vi "ProcessCANWrite.vi"(6 "Write Values":sgl[](array[numeric]), 8 "error in (no error)":errorcluster, 10 "Queue in":refnum<queue>, 11 "WriteFramesInfo":T1(array[cluster])) -> (0 "error out":errorcluster, 2 "WriteFramesSize":i32, 4 "Write Values":sgl[](array[numeric]))   [LabVIEW 2016, in "DSI-RT.lvlib"]
uses:
  DSI-RT.lvlib
  <vilib>/RioEmbeddedCAN/RioEmbeddedCAN.llb/CANFrameControl.ctl
  <vilib>/addons/Software Calibration Management/xSCM/Get/Get Variant.vi
  <vilib>/addons/Software Calibration Management/xSCM/SCM-API.lvlib
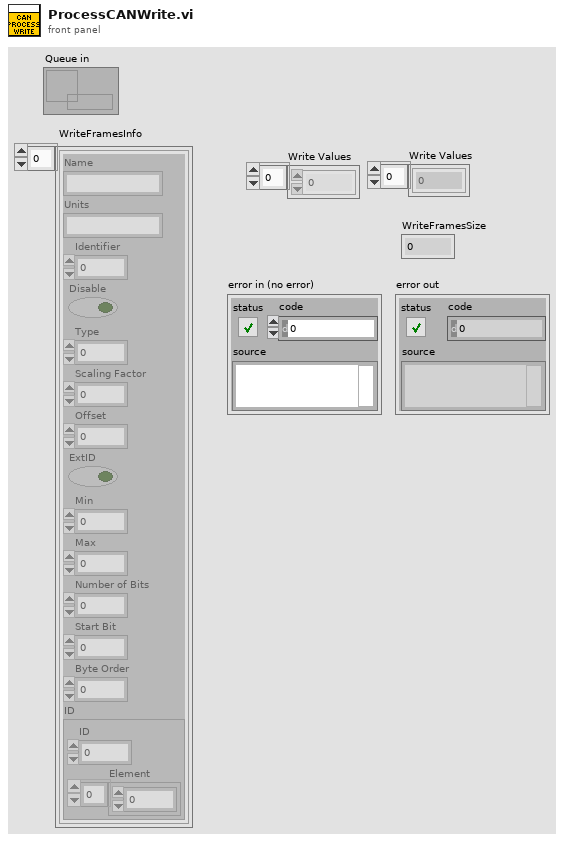
[diagram p1: front panel]
types:
  T1 = cluster{"Name":string, "Units":string, "Identifier":u32, "Disable":bool, "Type":u16, "Scaling Factor":sgl, "Offset":sgl, "ExtID":bool, "Min":sgl, "Max":sgl, "Number of Bits":u8, "Start Bit":u8, "Byte Order":u8, "ID":cluster{"ID":u32, "Element":i32[]}}[]
  T2 = cluster{"StartBit":u8, "Num Bits":u8, "Byte Order":u8, "Data Type":u8}
  T3 = cluster{"ScalingFactor":sgl, "Offset":sgl, "Maximum":sgl, "Minimum":sgl}
  T4 = typedef "CANFrameControl.ctl" = cluster{"identifier":u32, "extended?":bool, "type":u8, "payload":u8[]}
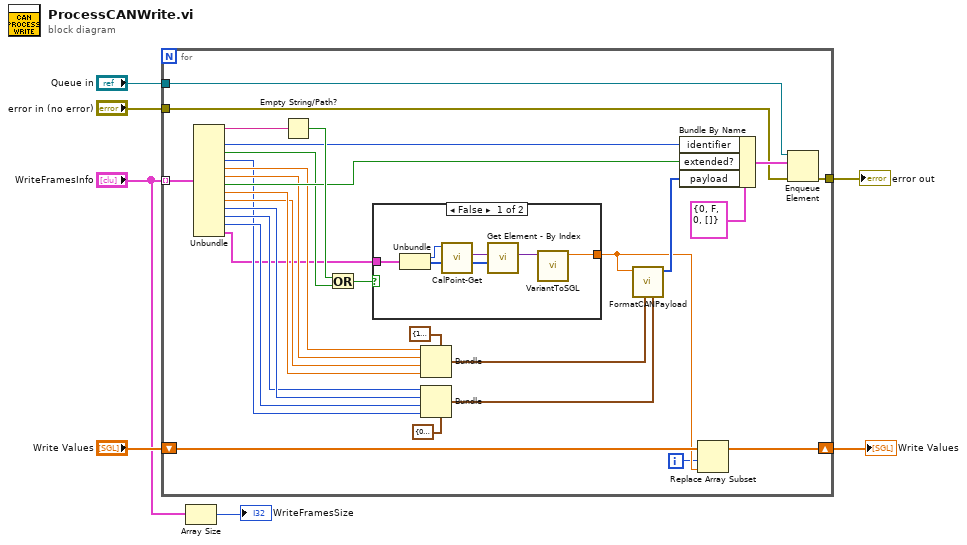
[diagram p0: block diagram]
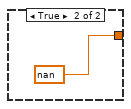
[diagram p2: hidden frame]
diagram:
  n1 = for {
    tunnel: "Queue in" -> [w34]
    shift-right: [w31] -> w5
    shift-left: "Write Values" -> [w33]
    tunnel: "WriteFramesInfo" -> [w24] mode=indexing
    tunnel: "error in (no error)" -> [w9]
    tunnel: [w8] -> w1
    i -> [w10]
    n2 = Unbundle(w24) -> ("Name"=w20:string, "Identifier"=w23:u32, "Disable"=w21:bool, "Type"=w12:u16, "Scaling Factor"=w19:sgl, "Offset"=w18:sgl, "ExtID"=w22:bool, "Min"=w17:sgl, "Max"=w16:sgl, "Number of Bits"=w15:u8, "Start Bit"=w14:u8, "Byte Order"=w13:u8, "ID"=w11:cluster{"ID":u32, "Element":i32[]})  [unwired: 1 out]
    n3 = Empty String/Path?(string/path=w20) -> (empty?=w25:bool)
    n4 = Or(x=w25, y=w21) -> (x .or. y?=w26:bool)
    n5 = case shown="False" w26 {
      tunnel: [w38 sgl nan ("Value")] -> w32
      tunnel: w11 -> [w40 _]
      frame False {
        n6 = Unbundle(w40) -> ("ID"=w41:u32, "Element"=w43:i32[])
        n7 = call-poly <vilib>:"CalPoint-Get.vi"("ID"=w41) -> ("Data"=w42:variant)  [unwired: 10 in]
        n8 = call <vilib>:"Get Element - By Index.vi"("Elements"=w43, "Variant"=w42) -> ("Element"=w39:variant)  [unwired: 8 in, 1 out]
        n9 = call "VariantToSGL.vi"("Element"=w39) -> ("Numeric"=w38:sgl)  [unwired: 10 in]
      }
      frame True {
      }
    }
    n10 = Bundle(cluster=T3 {"ScalingFactor"=1.0, "Offset"=0.0, "Maximum"=1.0, "Minimum"=0.0} ("DataFormat"), "ScalingFactor"=w19, "Offset"=w18, "Maximum"=w16, "Minimum"=w17) -> (w27:T3)
    n11 = Bundle(cluster=T2 {"StartBit"=0, "Num Bits"=0, "Byte Order"=1, "Data Type"=1} ("ByteFormat"), "StartBit"=w14, "Num Bits"=w15, "Byte Order"=w13, "Data Type"=w12) -> (w28:T2)
    n12 = call "FormatCANPayload.vi"("ByteFormat"=w28, "DataFormat"=w27, "Value"=w32) -> ("payload"=w36:u8[])  [unwired: 8 in]
    n13 = Bundle By Name(cluster=T4 {"identifier"=0, "extended?"=FALSE, "type"=0, "payload"=[]} ("CAN frame"), "identifier"=w23, "extended?"=w22, "payload"=w36) -> (w35:T4)
    n14 = Replace Array Subset(array=w33, new element=w32, index=w10) -> (w31:sgl[])
    n15 = Enqueue Element(queue=w34, element=w35, error in (no error)=w9) -> (error out=w8:errorcluster)  [unwired: 1 in, 2 out]
  }
  "Write Values" <- w5
  "error out" <- w1
  n16 = Array Size(array="WriteFramesInfo") -> (size(s)=→"WriteFramesSize":i32)
